vi "Open Soft Panel.vi"(8 "error in (no error)":errorcluster, 10 "SubPanel Ref":i32, 11 "Instrument in":refnum<class "Instrument.lvclass">) -> (0 "error out":errorcluster, 3 "Instrument out":refnum<class "Instrument.lvclass">)   [LabVIEW 2015, in "Instrument.lvlib" / "Instrument.lvclass"]
doc: "This method, when available, will open an Instruments soft-panel, allowing for parallel operation and/or viewing of an instruments state."
uses:
  Instrument.lvclass
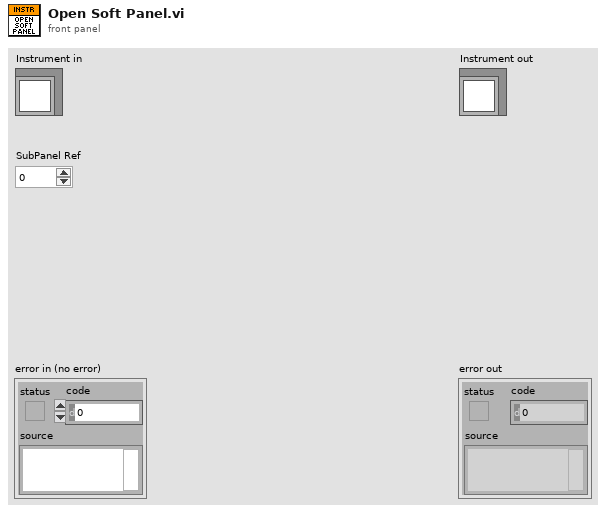
[diagram p1: front panel]
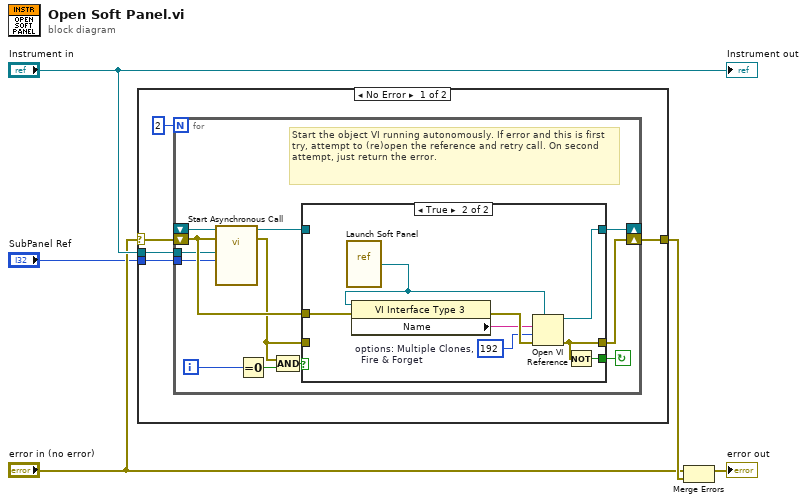
[diagram p0: block diagram]
diagram:
  n1 = case shown="No Error" "error in (no error)" {
    selector: "error in (no error)" -> [w7 w33]
    tunnel: "Instrument in" -> [w10 _]
    tunnel: [w8 w33] -> w3
    tunnel: "SubPanel Ref" -> [w6 _]
    frame No Error {
      n2 = for {
        N: 2 -> [_]
        tunnel: w10 -> [w21]
        shift-right: [w20] -> _
        shift-left: _ -> [w19]
        shift-right: [w17] -> w8
        shift-left: w7 -> [w22]
        tunnel: w6 -> [w11]
        i -> [w14]
        stop <- w12 continue-if-true
        # "Start the object VI running autonomously. If error and this is first try, attempt to (re)open the reference and retry call. On second attempt, just return the error."
        n3 = call-by-ref "Start Asynchronous Call"(reference=w19, error in=w22, "SubPanel Ref"=w11, "Instrument in"=w21) -> (reference out=w18:refnum<vi>, error out=w13:errorcluster)  [unwired: 8 in, 2 out]
        n4 = Equal To 0?(x=w14) -> (x = 0?=w15:bool)
        n5 = Compound Arithmetic op=AND(w13, w15) -> (w16:bool)
        n6 = case shown="True" w16 {
          tunnel: [w24 w29] -> w20
          tunnel: [w23 w27] -> w17
          tunnel: w18 -> [w24 _]
          tunnel: w13 -> [w23 _]
          tunnel: [_ w28] -> w12
          tunnel: w22 -> [_ w26]
          frame False {
          }
          frame True {
            w30 = 192  # options: Multiple Clones,   Fire & Forget
            n7 = vi-ref "Launch Soft Panel.vi"() -> (w25:refnum<vi>)
            n8 = property class="VI Interface Type 3"(reference=w25, error in=w26) -> (error out=w32:errorcluster, "Name"=w31:string)  [unwired: 1 out]
            n9 = Open VI Reference(type specifier VI Refnum (for type only)=w25, vi path=w31, options=w30, error in (no error)=w32) -> (vi reference=w29:refnum<vi>, error out=w27:errorcluster)  [unwired: 2 in]
            n10 = Not(x=w27) -> (.not. x?=w28:bool)
          }
        }
      }
    }
    frame Error {
    }
  }
  n11 = Merge Errors("error in (no error)", w3) -> (→"error out":errorcluster)
  "Instrument out" <- "Instrument in"
